vi "Generate Palette File List.vi"(8 "error in (no error)":errorcluster, 11 "Library Path":path) -> (0 "error out":errorcluster, 1 "Paths":path[](array[path]), 2 "List of Palette Files":T1[](array[typedef]), 3 "Library as Project item":refnum<vi>)   [LabVIEW 2018, in "Palette Generation.lvlib"]
doc: "This routine recurses through a library file and determines the virtual path of each project item and builds a list of virtual folders and their contents. This would be a whole lot easier if labview provided a ProjectItem property called virtual path...\n\nRetursn a list of project item real paths, virtual folders that will be used to construct Palette Files and the open project reference."
uses:
  Palette Generation.lvlib
  TypeDefs/Palette Fiole List.ctl
  <userlib>/_OpenG.lib/file/file.llb/Strip Path Extension - String__ogtk.vi
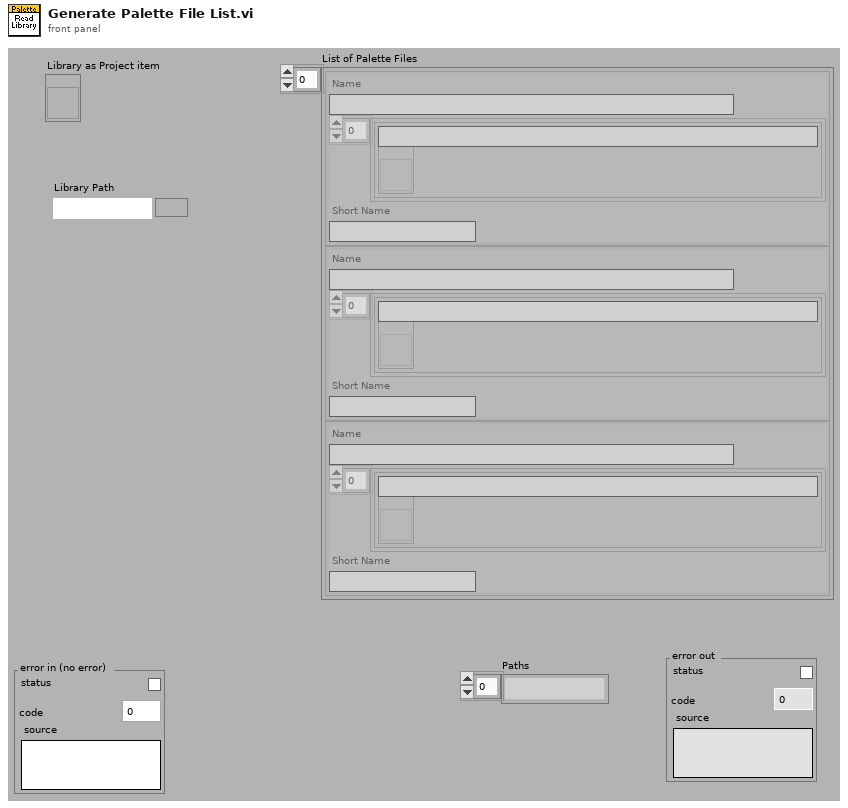
[diagram p1: front panel]
types:
  T1 = typedef "Palette Generation.lvlib/Palette Fiole List.ctl" = cluster{"Name":string, "Entries":cluster{string, refnum<vi>}[], "Short Name":string}
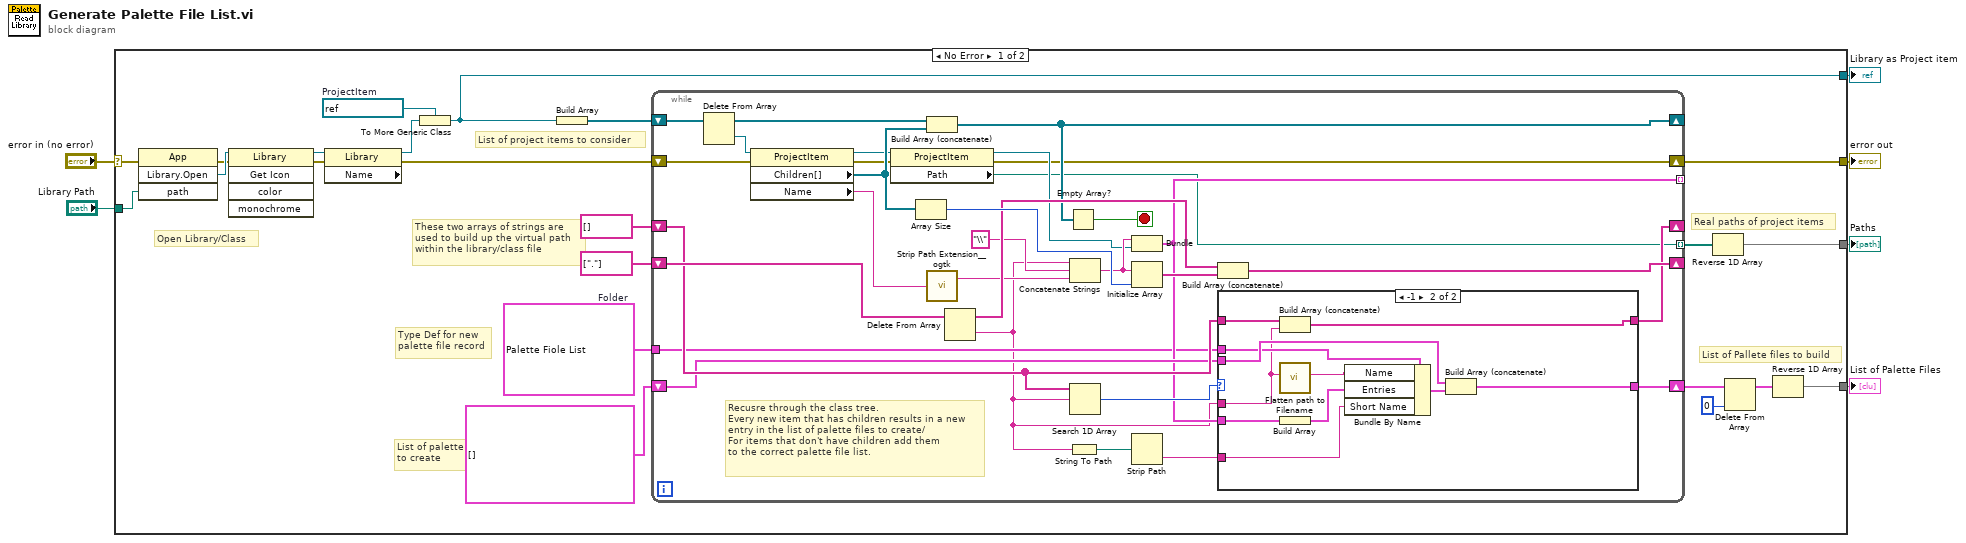
[diagram p0: block diagram]
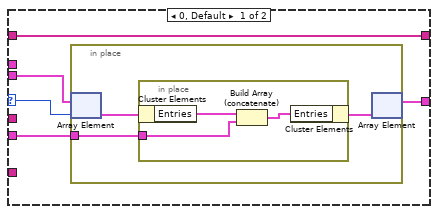
[diagram p2: hidden frame]
diagram:
  n1 = case shown="No Error" "error in (no error)" {
    selector: "error in (no error)" -> [w13 w82]
    tunnel: "Library Path" -> [w28 _]
    tunnel: [w12 _] -> w4
    tunnel: [w11 w82] -> w3
    tunnel: [w9 _] -> w2
    tunnel: [w8 _] -> w1
    frame No Error {
      w17 = T1 {"Name"="", "Entries"=[{".\\Registry\\Public\\Read Key Polymorphs\\Read Key-Value Template", refnum}, {".\\Registry\\Public\\Read Key Polymorphs\\Read Key-Value Variant", refnum}, {".\\Registry\\Public\\Read Key Polymorphs\\Read Key-Value Boolean Array", refnum}, {".\\Registry\\Public\\Read Key Polymorphs\\Read Key-Value VISA Ref", refnum}, {".\\Registry\\Public\\Read Key Polymorphs\\Read Key-Value Float Array", refnum}, {".\\Registry\\Public\\Read Key Polymorphs\\Read Key-Value String Dynamic", refnum}, {".\\Registry\\Public\\Read Key Polymorphs\\Read Key-Value Control", refnum}, {".\\Registry\\Public\\Read Key Polymorphs\\Read Key-Value Float", refnum}, {".\\Registry\\Public\\Read Key Polymorphs\\Read Key-Value Int32", refnum}, {".\\Registry\\Public\\Read Key Polymorphs\\Read Key-Value String", refnum}, {".\\Registry\\Public\\Read Key Polymorphs\\Read Key-Value Path", refnum}], "Short Name"=""}  # Folder
      w25 = refnum<vi> refnum  # ProjectItem
      # "List of Pallete files to build"
      # "Real paths of project items"
      # "These two arrays of strings are\nused to build up the virtual path\nwithin the library/class file"
      # "List of project items to consider"
      # "List of palette files\nto create"
      # "Type Def for new\npalette file record"
      # "Open Library/Class"
      n2 = invoke class="App" method="Library.Open"(error in=w13, "path"=w28) -> (error out=w23:errorcluster, "Open Library"=w27:refnum<vi>)  [unwired: 2 in, 2 out]
      n3 = invoke class="Library" method="Get Icon"(reference=w27, error in=w23) -> (reference out=w24:refnum<vi>, error out=w22:errorcluster)  [unwired: 3 in, 3 out]
      n4 = property class="Library" props=["Name"](reference=w24, error in=w22) -> (reference out=w26:refnum<vi>, error out=w19:errorcluster)  [unwired: 1 out]
      n5 = To More Generic Class(target class=w25, reference=w26) -> (generic class reference=w12:refnum<vi>)
      n6 = Build Array(w12) -> (w21:refnum<vi>[])
      n7 = while {
        shift-right: [w48] -> _
        shift-left: w21 -> [w59]
        shift-right: [w51] -> _
        shift-left: string[] ["."] -> [w57]
        tunnel: [w38] -> _ mode=indexing
        shift-right: [w30] -> w11
        shift-left: w19 -> [w44]
        shift-right: [w42] -> _
        shift-left: string[] [] -> [w41]
        shift-right: [w40] -> w7
        shift-left: T1[] [] -> [w39]
        tunnel: w17 -> [w37]
        tunnel: [w29] -> w10 mode=indexing
        stop <- w47 stop-if-true
        # "Recusre through the class tree.\nEvery new item that has children results in a new\nentry in the list of palette files to create/\nFor items that don't have children add them\nto the correct palette file list."
        n8 = Delete From Array(array=w59) -> (deleted portion=w58:refnum<vi>, array with subset deleted=w54:refnum<vi>[])  [unwired: 2 in]
        n9 = property class="ProjectItem"(reference=w58, error in=w44) -> (reference out=w49:refnum<vi>, error out=w31:errorcluster, "Children[]"=w53:refnum<vi>[], "Name"=w56:string)
        n10 = property class="ProjectItem"(reference=w49, error in=w31) -> (reference out=w32:refnum<vi>, error out=w30:errorcluster, "Path"=w29:path)
        n11 = Array Size(array=w53) -> (size(s)=w55:i32)
        n12 = Build Array (concatenate)(w54, w53) -> (w48:refnum<vi>[])
        n13 = call-poly <userlib>:"Strip Path Extension__ogtk.vi"("path"=w56) -> ("root"=w36:string)  [unwired: 1 out]
        n14 = Delete From Array(array=w57) -> (deleted portion=w35:string, array with subset deleted=w50:string[])  [unwired: 2 in]
        n15 = Empty Array?(array=w48) -> (empty?=w47:bool)
        n16 = String To Path(string=w35) -> (path=w34:path)
        n17 = Concatenate Strings(w35, "\\" ("string"), w36) -> (w46:string)
        n18 = Search 1D Array(1D array=w41, element=w35) -> (index of element=w43:i32)  [unwired: 1 out]
        n19 = Bundle(w46, w32) -> (w38:cluster{string, refnum<vi>})  [unwired: 1 out]
        n20 = Initialize Array(w46, w55) -> (w52:string[])
        n21 = Strip Path(path=w34) -> (name=w33:string)  [unwired: 1 out]
        n22 = Build Array (concatenate)(w50, w52) -> (w51:string[])
        n23 = case shown="-1" w43 {
          selector: w43 -> [w62 _]
          tunnel: w35 -> [_ w73]
          tunnel: [w64 w81] -> w42
          tunnel: w41 -> [w64 w80]
          tunnel: [w61 w79] -> w40
          tunnel: w39 -> [w63 w78]
          tunnel: w38 -> [w60 w77]
          tunnel: w37 -> [_ w76]
          tunnel: w33 -> [_ w71]
          frame 0, Default {
            n24 = in-place {
              in-place-border: w60 -> [w65]
              n25 = in-place-array #1(w63, w62) -> (w67:T1)
              n26 = in-place {
                in-place-border: w65 -> [w68]
                n27 = in-place-cluster #2(w67) -> ("Entries"=w70:cluster{string, refnum<vi>}[])
                n28 = Build Array (concatenate)(w70, w68) -> (w69:cluster{string, refnum<vi>}[])
                n29 = in-place-cluster #2("Entries"=w69) -> (w66:T1)
              }
              n30 = in-place-array #1(w66) -> (w61:T1[])  [unwired: 1 out]
            }
          }
          frame -1 {
            n31 = Build Array (concatenate)(w80, w73) -> (w81:string[])
            n32 = call "Flatten path to Filename.vi"("Virtual Folder's Virtual Path"=w73) -> ("result string"=w72:string)  [unwired: 2 in, 7 out]
            n33 = Build Array(w77) -> (w74:cluster{string, refnum<vi>}[])
            n34 = Bundle By Name(cluster=w76, "Name"=w72, "Entries"=w74, "Short Name"=w71) -> (w75:T1)
            n35 = Build Array (concatenate)(w78, w75) -> (w79:T1[])
          }
        }
      }
      n36 = Reverse 1D Array(array=w10) -> (reversed array=w8:path[])
      n37 = Delete From Array(array=w7, index=0) -> (array with subset deleted=w15:T1[])  [unwired: 1 in, 1 out]
      n38 = Reverse 1D Array(array=w15) -> (reversed array=w9:T1[])
    }
    frame Error {
    }
  }
  "List of Palette Files" <- w2
  "error out" <- w3
  "Library as Project item" <- w4
  "Paths" <- w1
